vi "WriteValue_Control2.vi"(9 "value":T1, 11 "reference":refnum<vi>) -> ()   [LabVIEW 2012]
uses:
  Typedefs/Control 2.ctl
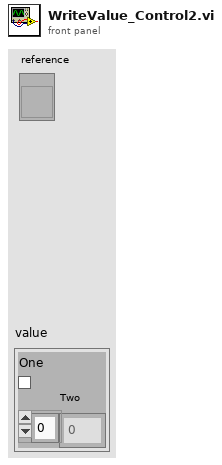
[diagram p1: front panel]
types:
  T1 = typedef "Control 2.ctl" = cluster{"One":bool, "Two":i32[]}
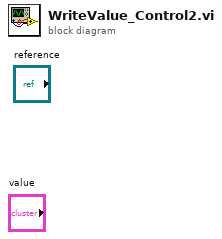
[diagram p0: block diagram]
diagram:
